vi "ApportionFlows.vi"(2 "Q[Total]:(l/min)":dbl, 4 "C:(%)":dbl, 8 "Temp (C)":dbl, 10 "Press (mBar)":dbl) -> (14 "Q[N2]:(l/min)":dbl, 15 "Rho[N2]:(kg/l)":dbl, 16 "Mdot[N2]:(g/min)":dbl, 17 "Q[Ethane]:(l/min)":dbl, 18 "Rho[Ethane]:(kg/l)":dbl, 19 "Mdot[Ethane]:(g/min)":dbl)   [LabVIEW 2021]
uses:
  Anemometry/Anemometry Sub Vis/Controls/GasCombo.ctl
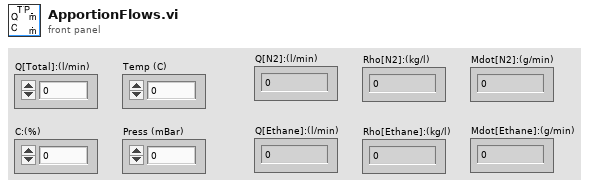
[diagram p1: front panel]
types:
  T1 = typedef "GasCombo.ctl" = string
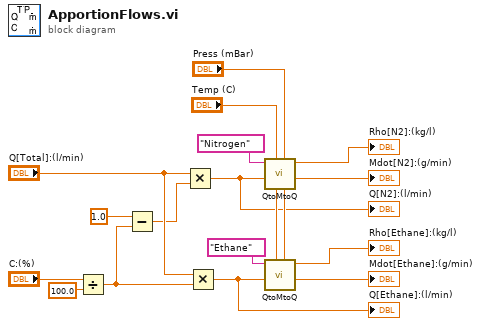
[diagram p0: block diagram]
diagram:
  n1 = Divide(x="C:(%)", y=100.0) -> (x/y=w3:dbl)
  n2 = Subtract(x=1.0, y=w3) -> (x-y=w4:dbl)
  n3 = Multiply(x="Q[Total]:(l/min)", y=w4) -> (x*y=w7:dbl)
  "Q[N2]:(l/min)" <- w7
  n4 = Multiply(x="Q[Total]:(l/min)", y=w3) -> (x*y=w5:dbl)
  "Q[Ethane]:(l/min)" <- w5
  n5 = call "QtoMtoQ.vi"("Pressure"="Press (mBar)", "Temperature"="Temp (C)", "Q in (l/min)"=w7, "Gas"=T1 "Nitrogen") -> ("Mdot out (g/min)"=→"Mdot[N2]:(g/min)":dbl, "Density (kg/m^3)(= g/l)"=→"Rho[N2]:(kg/l)":dbl)  [unwired: 3 in, 1 out]
  n6 = call "QtoMtoQ.vi"("Pressure"="Press (mBar)", "Temperature"="Temp (C)", "Q in (l/min)"=w5, "Gas"=T1 "Ethane") -> ("Mdot out (g/min)"=→"Mdot[Ethane]:(g/min)":dbl, "Density (kg/m^3)(= g/l)"=→"Rho[Ethane]:(kg/l)":dbl)  [unwired: 3 in, 1 out]
